vi "QueryACCcurrent.vi"(5 "COM Port":refnum<visa-resource-name>="COM6") -> (1 "ACC":dbl(slide) min=0.0 max=90.0 scale=0.0..90.0)   [LabVIEW 2020]
uses:
  <vilib>/Instr/_visa.llb/VISA Configure Serial Port (Instr).vi
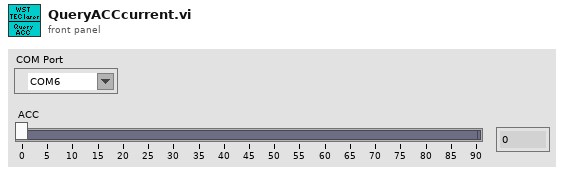
[diagram p1: front panel]
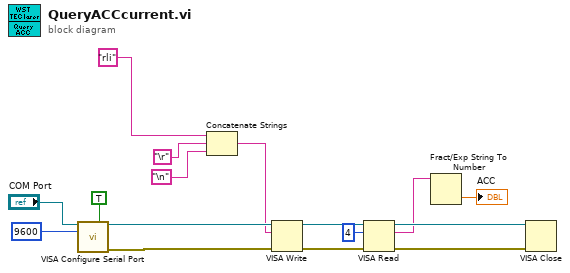
[diagram p0: block diagram]
diagram:
  n1 = call-poly "VISA Configure Serial Port"("VISA resource name"="COM Port", "Enable Termination\nChar (T)"=TRUE ("Enable Termination\nChar (T)"), "baud rate (9600)"=u32 9600) -> ("VISA resource name out"=w13:refnum<visa-resource-name>, "error out"=w12:errorcluster)  [unwired: 11 in]
  n2 = Concatenate Strings("rli", "\r", "\n") -> (w9:string)
  n3 = VISA Write(VISA resource name=w13, write buffer=w9, error in (no error)=w12) -> (VISA resource name out=w7:refnum<visa-resource-name>, error out=w6:errorcluster)  [unwired: 1 out]
  n4 = VISA Read(VISA resource name=w7, byte count=u32 4, error in (no error)=w6) -> (VISA resource name out=w5:refnum<visa-resource-name>, read buffer=w2:string, error out=w4:errorcluster)  [unwired: 1 out]
  n5 = Fract/Exp String To Number(string=w2) -> (number=→"ACC":dbl)  [unwired: 3 in, 1 out]
  n6 = VISA Close(VISA resource name=w5, error in (no error)=w4) -> ()  [unwired: 1 out]
